vi "Day 01 Part 1.vi"(11 "Input":string) -> (3 "Output":i16)   [LabVIEW 2021]
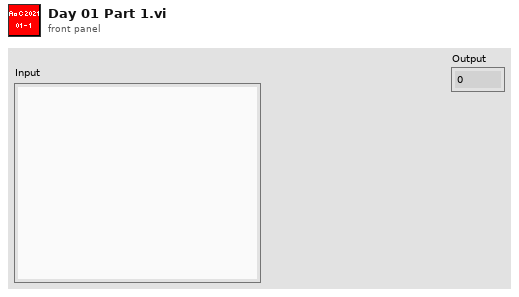
[diagram p1: front panel]
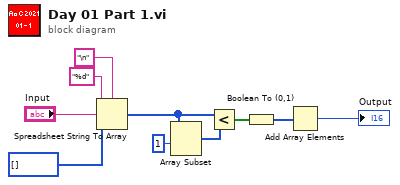
[diagram p0: block diagram]
diagram:
  n1 = Spreadsheet String To Array(delimiter (Tab)="\n", format string="%d", spreadsheet string="Input", array type (2D Dbl)=i32[] []) -> (array=w2:i32[])
  n2 = Array Subset(array=w2, index=1 ("length")) -> (w6:i32[])  [unwired: 1 in]
  n3 = Less?(x=w2, y=w6) -> (x < y?=w8:bool[])
  n4 = Boolean To (0,1)(Boolean=w8) -> (0, 1=w10:i16[])
  n5 = Add Array Elements(numeric array=w10) -> (sum=→"Output":i16)
